vi "Set_Error.vi"(0 "CustomErrors":T1, 1 "SetError(True)":bool=TRUE, 2 "Description":string, 3 "Project Specific Error Code start range":i32=6700, 4 "Error SubVI Level(1)":i32=2, 5 "error in (no error)":errorcluster) -> (19 "error out":errorcluster)   [LabVIEW 2020, in "DP_WebView.lvclass"]
uses:
  DP_WebView.lvclass
  ctrls/ErrorCode.ctl
panel:
  in  "code (5000)":i32=5000
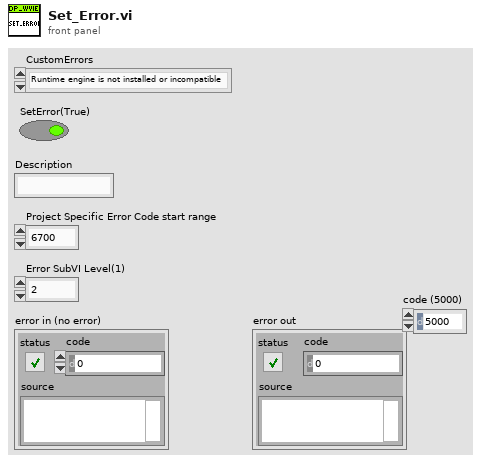
[diagram p1: front panel]
types:
  T1 = typedef "DP_WebView.lvclass/ErrorCode.ctl" = enum16{"Runtime engine is not installed or incompatible", "User Data Folder cannot be set", "Others", "JavaScript call failed", "PDF Printing Issue"}
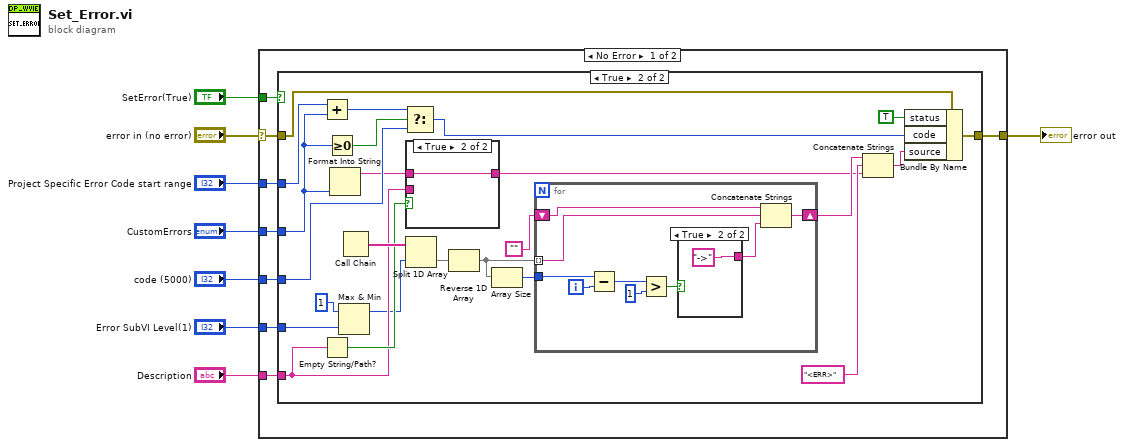
[diagram p0: block diagram]
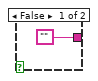
[diagram p4: hidden frame]
diagram:
  n1 = case shown="No Error" "error in (no error)" {
    selector: "error in (no error)" -> [w12 w55]
    tunnel: [w16 w55] -> w3
    tunnel: "SetError(True)" -> [w15 _]
    tunnel: "code (5000)" -> [w14 _]
    tunnel: "Description" -> [w13 _]
    tunnel: "Project Specific Error Code start range" -> [w11 _]
    tunnel: "Error SubVI Level(1)" -> [w10 _]
    tunnel: "CustomErrors" -> [w9 _]
    frame No Error {
      n2 = case shown="True" w15 {
        tunnel: w12 -> [w17 w41]
        tunnel: [w17 w40] -> w16
        tunnel: w14 -> [_ w30]
        tunnel: w13 -> [_ w24]
        tunnel: w11 -> [_ w23]
        tunnel: w10 -> [_ w21]
        tunnel: w9 -> [_ w19]
        frame False {
        }
        frame True {
          n3 = Add(x=w23, y=w19) -> (x+y=w28:i32)
          n4 = Empty String/Path?(string/path=w24) -> (empty?=w26:bool)
          n5 = Greater Or Equal To 0?(x=w19) -> (x >= 0?=w27:bool)
          n6 = Format Into String(w19) -> (resulting string=w18:string)  [unwired: 3 in, 1 out]
          n7 = Max & Min(x=1, y=w21) -> (max(x,y)=w20:i32)  [unwired: 1 out]
          n8 = Call Chain() -> (call chain=w38:string[])
          n9 = Select(t=w28, s=w27, f=w30) -> (s? t:f=w29:i32)
          n10 = case shown="True" w26 {
            tunnel: w18 -> [_ w43]
            tunnel: w24 -> [w42 _]
            tunnel: [w42 w43] -> w25
            frame False {
            }
            frame True {
            }
          }
          n11 = Split 1D Array(array=w38, index=w20) -> (second subarray=w37:string[])  [unwired: 1 out]
          n12 = Reverse 1D Array(array=w37) -> (reversed array=w31:string[])
          n13 = Array Size(array=w31) -> (size(s)=w36:i32)
          n14 = for {
            shift-right: [w44] -> w34
            shift-left: "" -> [w47]
            tunnel: w31 -> [w45] mode=indexing
            tunnel: w36 -> [w52]
            i -> [w51]
            n15 = Subtract(x=w52, y=w51) -> (x-y=w50:i32)
            n16 = Greater?(x=w50, y=1) -> (0:w48:bool)
            n17 = case shown="True" w48 {
              tunnel: ["" "->"] -> w46
              frame False {
              }
              frame True {
              }
            }
            n18 = Concatenate Strings(w47, w45, w46) -> (w44:string)
          }
          n19 = Concatenate Strings(w34, "<ERR>" ("Substring"), w25) -> (w35:string)
          n20 = Bundle By Name(cluster=w41, "status"=TRUE ("Bundle Element"), "code"=w29, "source"=w35) -> (w40:errorcluster)
        }
      }
    }
    frame Error {
    }
  }
  "error out" <- w3
